vi "SCM Init.vi"() -> (0 "error out":errorcluster)   [LabVIEW 2010]
uses:
  TPS Global.vi
  SCM Global.vi
  <vilib>/Utility/config.llb/NI_LVConfig.lvlib
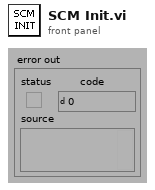
[diagram p1: front panel]
types:
  T1 = cluster{"Board":i32, "Channel":i32, "Range":i32, "Interval":i32, "Offset":dbl, "Multiplier":dbl, "Field":string, "Name":string}
  T2 = typedef "NI_LVConfig.lvlib/Config Data RefNum.ctl" = refnum<k1>
  T3 = cluster{"Board":i32, "Channel":i32, "Range":i32, "Interval":i32, "Offset":dbl, "Multiplier":dbl, "Field":string, "Name":string}[]
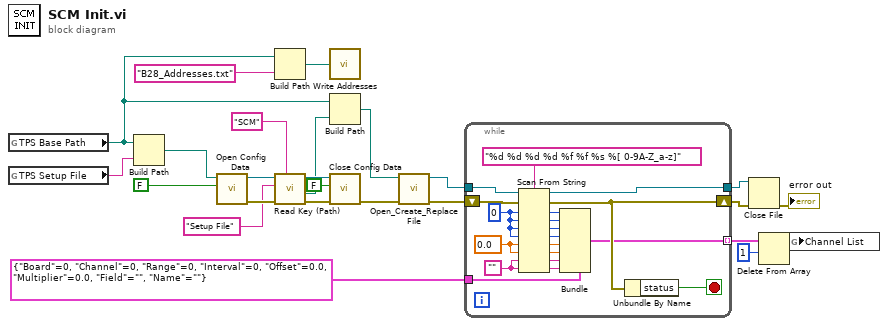
[diagram p0: block diagram]
diagram:
  n1 = global read "TPS Global.vi" "TPS Base Path"() -> (w4:path)
  n2 = global read "TPS Global.vi" "TPS Setup File"() -> (w6:string)
  n3 = Build Path(base path=w4, name or relative path=w6) -> (appended path=w15:path)
  n4 = call <vilib>:"Open Config Data.vi"("create file if necessary (T)"=FALSE ("create file if necessary? (T)"), "configuration file path"=w15) -> ("error out"=w13:errorcluster, "refnum"=w12:T2)  [unwired: 7 in, 1 out]
  n5 = Build Path(base path=w4, name or relative path="B28_Addresses.txt") -> (appended path=w2:path)
  n6 = call <vilib>:"Read Key (Path).vi"("section"="SCM", "error in (no error)"=w13, "key"="Setup File", "refnum"=w12) -> ("error out"=w10:errorcluster, "value"=w7:path, "refnum out"=w11:T2)  [unwired: 4 in, 1 out]
  n7 = call "Write Addresses.vi"("Address File"=w2) -> ()
  n8 = Build Path(base path=w4, name or relative path=w7) -> (appended path=w17:path)
  n9 = call <vilib>:"Close Config Data.vi"("error in (no error)"=w10, "write file if changed (T)"=FALSE, "refnum"=w11) -> ("error out"=w16:errorcluster)  [unwired: 7 in, 1 out]
  n10 = call <vilib>:"Open_Create_Replace File.vi"("error in (no error)"=w16, "file path"=w17) -> ("error out"=w18:errorcluster, "refnum"=w19:refnum<file>)  [unwired: 6 in, 2 out]
  n11 = while {
    shift-right: [w42] -> w21
    shift-left: w18 -> [w44]
    tunnel: w19 -> [w40]
    tunnel: [w39] -> w20
    tunnel: T1 {"Board"=0, "Channel"=0, "Range"=0, "Interval"=0, "Offset"=0.0, "Multiplier"=0.0, "Field"="", "Name"=""} -> [w34]
    tunnel: [w37] -> w24 mode=indexing
    stop <- w41 stop-if-true
    w28 = 0.0
    w26 = ""
    w43 = 0
    n12 = Scan From String("%d %d %d %d %f %f %s %[ 0-9A-Z_a-z]" ("format string"), w40, w44, default 1=w43, default 2=w43, default 3=w43, default 4=w43, default 5=w28, default 6=w28, default 7=w26, default 8=w26) -> (w39:refnum<file>, w42:errorcluster, output 1=w36:i32, output 2=w35:i32, output 3=w33:i32, output 4=w32:i32, output 5=w31:dbl, output 6=w30:dbl, output 7=w29:string, output 8=w27:string)
    n13 = Bundle(cluster=w34, "Board"=w36, "Channel"=w35, "Range"=w33, "Interval"=w32, "Offset"=w31, "Multiplier"=w30, "Field"=w29, "Name"=w27) -> (w37:T1)
    n14 = Unbundle By Name(w42) -> ("status"=w41:bool)
  }
  n15 = Close File(refnum=w20, error in=w21) -> (error out=→"error out":errorcluster)  [unwired: 1 out]
  n16 = Delete From Array(array=w24, length=1) -> (array with subset deleted=w25:T3)  [unwired: 1 in, 1 out]
  n17 = global write "SCM Global.vi" "Channel List"(w25) -> ()
